vi "FTW-Endpoint-Symbols.vi"() -> ()   [LabVIEW 2013, in "FTW-Actor-Endpoint.lvclass"]
uses:
  FTW-Actor-Endpoint.lvclass
panel:
  out "Symbols":T1(array[cluster]) {"Symbol Value" format="0x%08x  (%d)"}
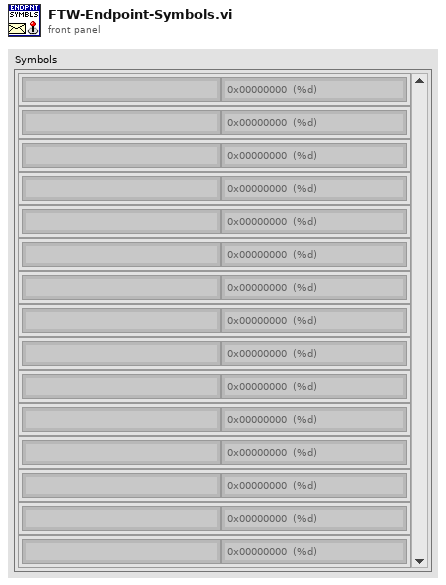
[diagram p1: front panel]
types:
  T1 = cluster{"Symbol Name":string, "Symbol Value":i32}[]
diagram:
